vi "data_read.vi"(8 "error in (no error)":errorcluster, 10 "dataContainer":variant, 11 "ini_file_refnum":T1) -> (0 "error out":errorcluster, 2 "dataValue":variant, 3 "ini_file_refnum_out":T1)   [LabVIEW 2015, in "ini_work_Library.lvlib"]
doc: "Created by Artem Shevelev\nshevelev.pro\nartem@shevelev.pro\nLabVIEW Portal: https://labviewportal.org/memberlist.php?mode=viewprofile&u=2340"
uses:
  ini_work_Library.lvlib
  <vilib>/Utility/config.llb/Config Data RefNum.ctl
  <vilib>/Utility/config.llb/NI_LVConfig.lvlib
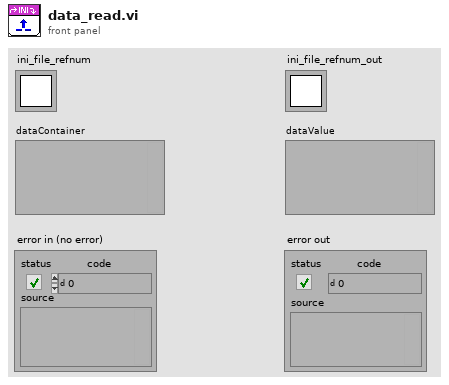
[diagram p1: front panel]
types:
  T1 = typedef "NI_LVConfig.lvlib/Config Data RefNum.ctl" = refnum<k1>
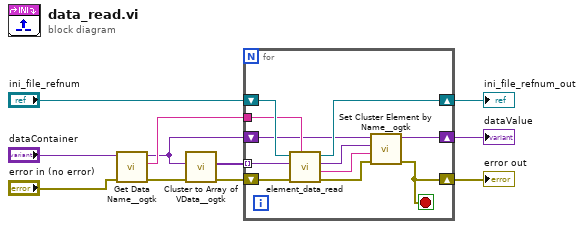
[diagram p0: block diagram]
diagram:
  n1 = call <userlib>:"Get Data Name__ogtk.vi"("error in (no error)"="error in (no error)", "Data"="dataContainer") -> ("error out"=w7:errorcluster, "Data Name"=w5:string, "Data dup"=w2:variant)  [unwired: 7 in]
  n2 = call <userlib>:"Cluster to Array of VData__ogtk.vi"("error in (no error)"=w7, "Cluster"=w2) -> ("error out"=w10:errorcluster, "Array of VData"=w11:variant[])  [unwired: 8 in]
  n3 = for {
    tunnel: w11 -> [w18] mode=indexing
    shift-right: [w12] -> w3
    shift-left: w10 -> [w21]
    shift-right: [w20] -> w4
    shift-left: "ini_file_refnum" -> [w22]
    tunnel: w5 -> [w19]
    shift-right: [w14] -> w1
    shift-left: w2 -> [w17]
    stop <- w12 stop-if-true
    n4 = call "element_data_read.vi"("container_name"=w19, "error in (no error)"=w21, "data_type"=w18, "Refnum in"=w22) -> ("error out"=w13:errorcluster, "Data Name"=w15:string, "data_out"=w16:variant, "Refnum out"=w20:T1)  [unwired: 4 in]
    n5 = call <userlib>:"Set Cluster Element by Name__ogtk.vi"("error in (no error)"=w13, "Element Name (\"\": New Element Data Name)"=w15, "New Element Value"=w16, "Cluster"=w17) -> ("error out"=w12:errorcluster, "VCluster out"=w14:variant)  [unwired: 5 in, 1 out]
  }
  "ini_file_refnum_out" <- w4
  "error out" <- w3
  "dataValue" <- w1
